vi "Catch Process Error.vi"(10 "Process Error":errorcluster, 11 "SMO":refnum<class "SMO.lvclass">) -> (0 "error out":errorcluster, 3 "SMO out":refnum<class "SMO.lvclass">)   [LabVIEW 2021, in "smo.lvlib" / "SMO.lvclass"]
uses:
  SMO.lvclass
  SMO.lvclass/SMO.ctl
panel:
  # "For instructions on how to use the JKI State Machine Objects, examples and video tutorials, visit:\nhttp://jki.net/state-machine-objects/\n\nJKI State Machine Objects™\nhttp://jki.net/state-machine-objects/\nCopyright (C) 2005-2015, JKI <info@jki.net>\nALL RIGHTS RESERVED"
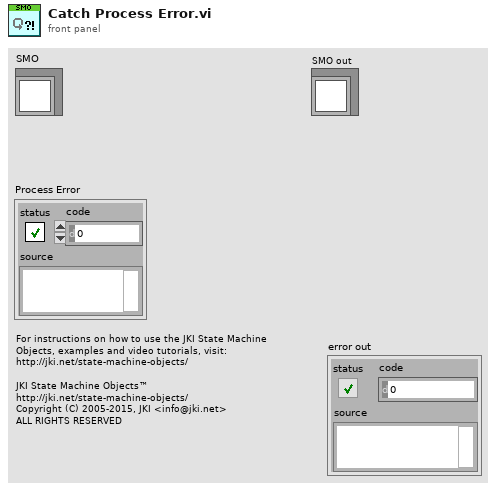
[diagram p1: front panel]
types:
  T1 = typedef "smo.lvlib/SMO.lvclass/PrivateData--Ref.ctl" = refnum<data-value>
  T2 = typedef "smo.lvlib/SMO.lvclass/PrivateData--Cluster.ctl" = cluster{"Parent Call":T3, "Registered Processes":T4[], "Sync Notifier":refnum<notifier>, "Process Error Notifier":refnum<notifier>, "Protected Events":T5, "Public Events":T6, "SMO State":T7, "[Attributes]":variant, "Launcher Close":refnum<notifier>, "Caller Watchdog":refnum<queue>, "Accessibility":T8, "NbStaticDependencies":u32}
  T3 = typedef "smo.lvlib/SMO.lvclass/Parent Call--Enum.ctl" = enum16{"Allows parent to run", "Does not request parent to run"}
  T4 = typedef "smo.lvlib/SMO.lvclass/RegisteredProcessData--Cluster.ctl" = cluster{"Name":string, "Static VI Ref":refnum<vi>, "Running":bool, "NotifierRef":u32}
  T5 = typedef "smo.lvlib/SMO.lvclass/Protected Events.ctl" = cluster{"StopProcesses":refnum<user-event>, "AbortProcesses":refnum<user-event>, "Config Changed":refnum<user-event>, "Dependency":refnum<user-event>}
  T6 = typedef "smo.lvlib/SMO.lvclass/Public Events.ctl" = cluster{"Error":refnum<user-event>, "State":refnum<user-event>, "Reserve State":refnum<user-event>}
  T7 = typedef "smo.lvlib/SMO.lvclass/SMOState --Enum.ctl" = enum16{"unknown", "Created", "Started", "Stopped"}
  T8 = typedef "smo.lvlib/SMO.lvclass/Accessibility--Cluster.ctl" = cluster{"Lock Key":string, "Reserve State":T9}
  T9 = typedef "smo.lvlib/SMO.lvclass/Reserve State--Enum.ctl" = enum16{"Unreserved", "Reserved", "Self-locked"}
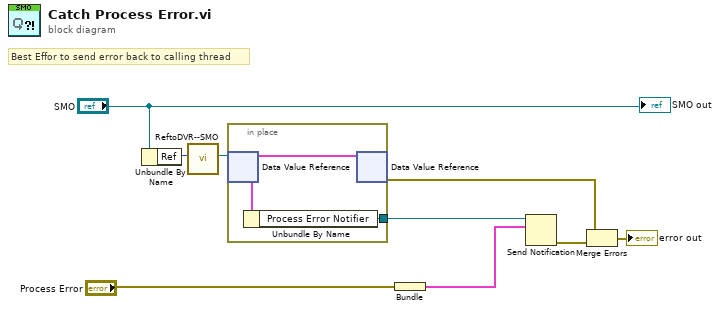
[diagram p0: block diagram]
diagram:
  # "Best Effor to send error back to calling thread"
  n1 = Unbundle By Name("SMO") -> ("Ref"=w3:u32)
  n2 = call "ReftoDVR--SMO.vi"("Ref"=w3) -> ("Ref"=w2:T1)  [unwired: 10 in]
  n3 = in-place {
    in-place-border: [w11] -> w9
    n4 = in-place-dvr #1(w2) -> (w10:T2)  [unwired: 1 out]
    n5 = Unbundle By Name(w10) -> ("Process Error Notifier"=w11:refnum<notifier>)
    n6 = in-place-dvr #1(w10) -> (w5:errorcluster)  [unwired: 1 out]
  }
  n7 = Bundle("Process Error"="Process Error") -> (w7:cluster{"Process Error":errorcluster})  [unwired: 1 in]
  n8 = Send Notification(notification=w7, notifier=w9) -> (error out=w6:errorcluster)  [unwired: 1 in, 1 out]
  n9 = Merge Errors(w5, w6) -> (→"error out":errorcluster)
  "SMO out" <- "SMO"
